vi "amplified signal.vi"() -> ()   [LabVIEW 2017]
panel:
  out "main signal":waveform(dbl)[](graph)
  out "amplified signal":waveform(dbl)(graph)
  out "x*y":dbl[](array[numeric])
  in  "path 3":path
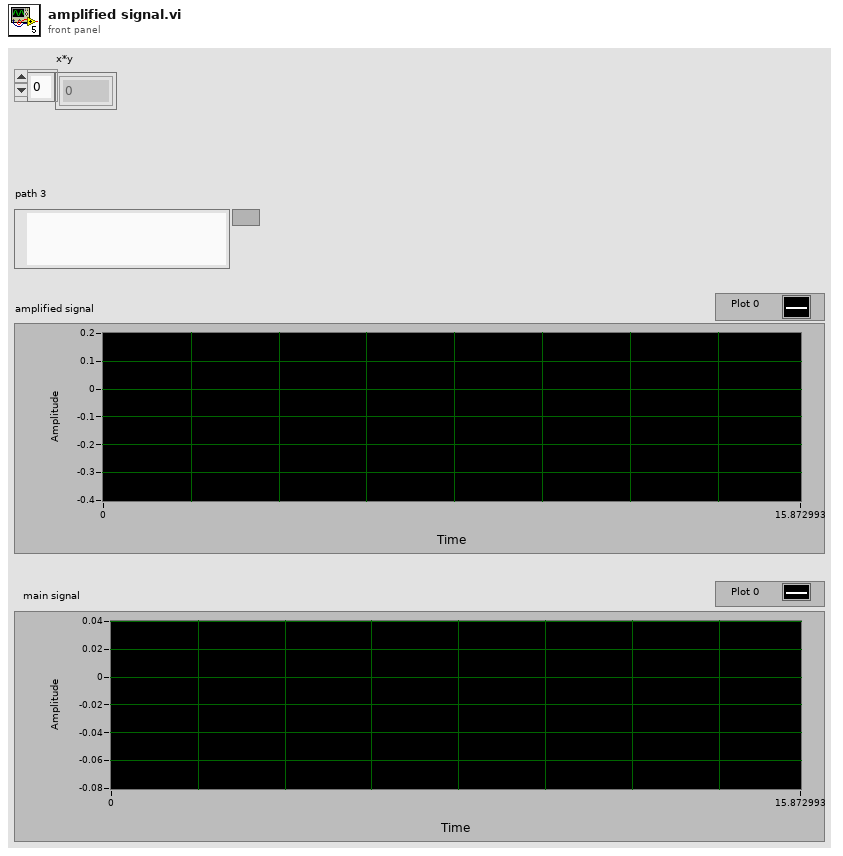
[diagram p1: front panel]
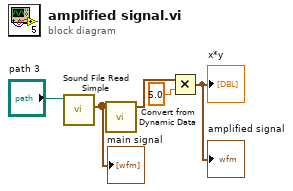
[diagram p0: block diagram]
diagram:
  n1 = call <vilib>:"Sound File Read Simple.vi"("path"="path 3") -> ("data"=w4:waveform(dbl)[])  [unwired: 7 in, 3 out]
  "main signal" <- w4
  n2 = call "Convert from Dynamic Data"("Dynamic Data Type"=w4) -> ("Waveform"=w3:waveform(dbl))  [unwired: 3 in]
  n3 = Multiply(x=w3, y=5.0) -> (x*y=→"x*y" →"amplified signal":waveform(dbl))
